vi "Initialise_puffer.vi"() -> (5 "Plug in titles":string[](array[string]), 7 "Plug in values":string[](array[string]))   [LabVIEW 2010]
uses:
  Controls/Post_Process.ctl
  ADAM Client/Sub VIs/ADAM Controls/Update_scan_value.ctl
  Globals/Meas_global.vi
  Globals/Extra_Commands_Global.vi
  Globals/Trav_pos_global.vi
  Globals/Dynamic_call_global.ph.vi
  Globals/Constants_global.vi
panel:
  out "Case Currently On":string
  out "Pulse Length":dbl format="%.2f"
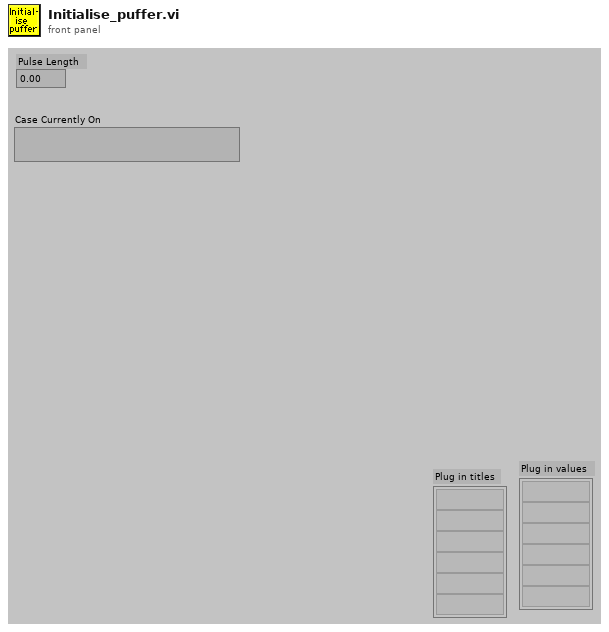
[diagram p1: front panel]
types:
  T1 = typedef "Post_Process.ctl" = enum16{"Take New Data", "Post Process Raw Data File"}
  T2 = typedef "Update_scan_value.ctl" = cluster{"Channel Name":string, "New Value":dbl}
  T3 = typedef "Traverse_cluster.ctl" = cluster{"Start X":dbl, "Start Y":dbl, "Start Z":dbl, "End X":dbl, "End Y":dbl, "End Z":dbl, "No. of pts.":i32, "Spacing":T4, "Filename":path, "Tunnel Speed":dbl, "Averaging time (min)":dbl, "Extra Commands":string, "Specific Arguments":string, "Emission Rate (l/min)":dbl, "Trace Gas Concentration (%)":dbl, "Density Ratio":string, "Comments":string, "Row No":i32, "Row Type Selector":T5, "Completion time":string, "Row Duration (mins)":dbl, "No. of Valid pts.":i32, "Meas Setup File":string}
  T4 = typedef "Spacing.ctl" = enum16{"Linear", "Log", "Gauss", "Specified", "N/A"}
  T5 = typedef "Multi_run_mode.ctl" = enum16{"Move Traverse Only", "Set Tunnel Speed Only", "Set Source Only", "Set Measurement Conditions", "Single Measurement", "Vertical Profile", "Lateral Profile", "Longitudinal Profile", "Explore Volume", "Multi-Axis Profile", "Auto Calibrate", "Meas Fast FID Bkgnd", "Check Beam Power", "Scanning Valve Measurement", "Run VI Named:", "Set ADAM Ch", "Wait (minutes)", "Send Message", "Synchronize With:", "Fall Back to this Row", "Turn Off Row Repeating", "Blank Row"}
  T6 = typedef "Rendezvous RefNum" = refnum<k1>
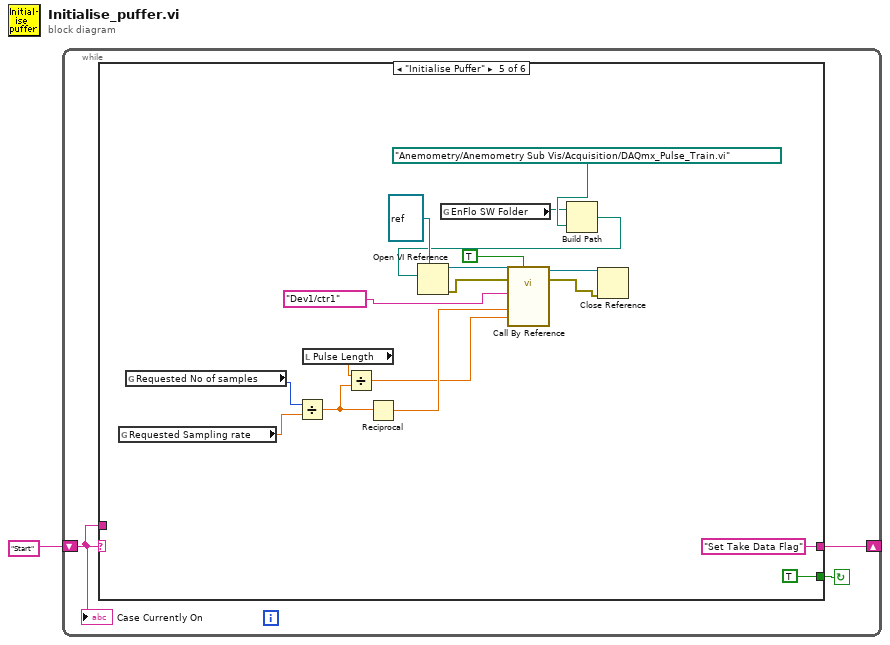
[diagram p0: block diagram]
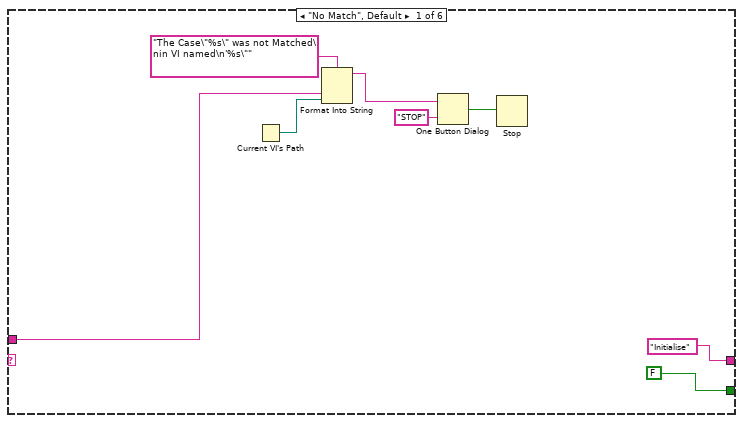
[diagram p2: hidden frame]
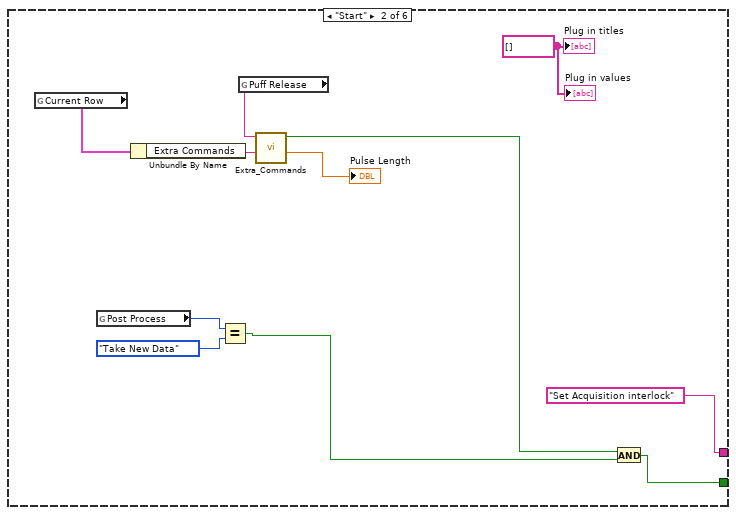
[diagram p3: hidden frame]
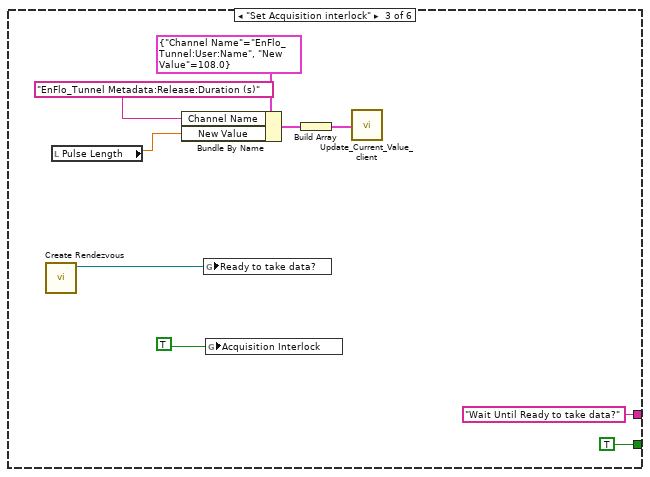
[diagram p4: hidden frame]
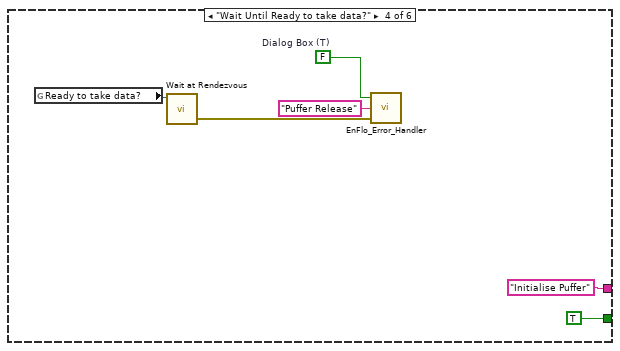
[diagram p5: hidden frame]
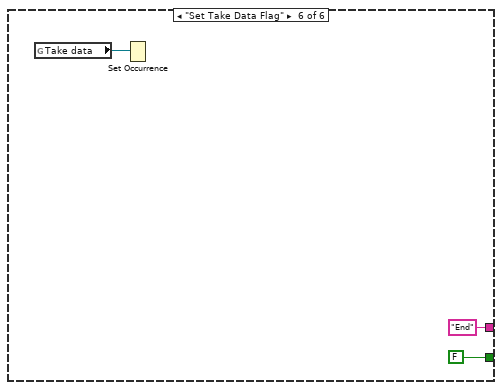
[diagram p6: hidden frame]
diagram:
  n1 = while {
    shift-left: "Start" -> [w2]
    shift-right: [w3] -> _
    stop <- w4 continue-if-true
    n2 = case shown="\"Initialise Puffer\"" w2 {
      tunnel: [FALSE w14 TRUE ("Command Found") TRUE ("Command Found") TRUE ("Command Found") FALSE ("Command Found")] -> w4
      tunnel: ["Initialise" "Set Acquisition interlock" "Wait Until Ready to take data?" "Initialise Puffer" "Set Take Data Flag" "End"] -> w3
      tunnel: w2 -> [w7 _ _ _ _ _]
      frame "No Match", Default {
        n3 = Current VI's Path() -> (path=w6:path)
        n4 = Format Into String(format string="The Case\"%s\" was not Matched\nin VI named\n'%s\"" ("Format String"), w7, w6) -> (resulting string=w10:string)  [unwired: 2 in, 1 out]
        n5 = One Button Dialog(message=w10, button name ("OK")="STOP") -> (true=w8:bool)
        n6 = Stop(stop? (T)=w8) -> ()
      }
      frame "Start" {
        w13 = string[] [] ("Plug in titles")
        n7 = global read "Trav_pos_global.vi" "Current Row"() -> (w23:T3)
        n8 = global read "Meas_global.vi" "Post Process"() -> (w17:T1)
        n9 = Unbundle By Name(w23) -> ("Extra Commands"=w21:string)
        n10 = Equal?(x=w17, y=Post_Process."Take New Data" ("Post Process")) -> (x = y?=w15:bool)
        n11 = global read "Extra_Commands_Global.vi" "Puff Release"() -> (w22:string)
        n12 = call "Extra_Commands.vi"("String to Search"=w21, "Command"=w22) -> ("Numeric Value"=→"Pulse Length":dbl, "Command Found"=w16:bool)  [unwired: 2 in, 2 out]
        n13 = And(x=w16, y=w15) -> (x .and. y?=w14:bool)
        "Plug in values" <- w13
        "Plug in titles" <- w13
      }
      frame "Set Acquisition interlock" {
        n14 = call <vilib>:"Create Rendezvous.vi"() -> ("rendezvous"=w29:T6)  [unwired: 5 in, 2 out]
        n15 = local read "Pulse Length"() -> (w24:dbl)
        n16 = Bundle By Name(cluster=T2 {"Channel Name"="EnFlo_Tunnel:User:Name", "New Value"=108.0} ("Update Scan Value Cluster"), "Channel Name"="EnFlo_Tunnel Metadata:Release:Duration (s)", "New Value"=w24) -> (w27:T2)
        n17 = global write "Dynamic_call_global.ph.vi" "Ready to take data?"(w29) -> ()
        n18 = global write "Dynamic_call_global.ph.vi" "Acquisition Interlock"(TRUE ("Remote control")) -> ()
        n19 = Build Array(w27) -> (w26:T2[])
        n20 = call "Update_Current_Value_client.vi"("Update array in"=w26) -> ()  [unwired: 1 in]
      }
      frame "Wait Until Ready to take data?" {
        w34 = FALSE  # Dialog Box (T)
        n21 = global read "Dynamic_call_global.ph.vi" "Ready to take data?"() -> (w37:T6)
        n22 = call <vilib>:"Wait at Rendezvous.vi"("rendezvous"=w37) -> ("error out"=w35:errorcluster)  [unwired: 4 in, 2 out]
        n23 = call "EnFlo_Error_Handler.vi"("error in (no error)"=w35, "Error Type"="Puffer Release", "Dialog Box (T)"=w34) -> ()  [unwired: 3 out]
      }
      frame "Initialise Puffer" {
        n24 = global read "Meas_global.vi" "Requested Sampling rate"() -> (w54:dbl)
        n25 = global read "Meas_global.vi" "Requested No of samples"() -> (w55:i32)
        n26 = Divide(x=w55, y=w54) -> (x/y=w42:dbl)
        n27 = local read "Pulse Length"() -> (w41:dbl)
        n28 = Divide(x=w41, y=w42) -> (x/y=w40:dbl)
        n29 = Reciprocal(x=w42) -> (1/x=w43:dbl)
        n30 = global read "Constants_global.vi" "EnFlo SW Folder"() -> (w45:path)
        n31 = Build Path(base path=w45, name or relative path=path "Anemometry/Anemometry Sub Vis/Acquisition/DAQmx_Pulse_Train.vi") -> (appended path=w47:path)
        n32 = Open VI Reference(type specifier VI Refnum (for type only)=refnum<vi> refnum, vi path=w47) -> (vi reference=w48:refnum<vi>, error out=w51:errorcluster)  [unwired: 4 in]
        n33 = call-by-ref "?"(reference=w48, error in=w51, "Counter(s)"=tag "Dev1/ctr1", "Start?"=TRUE, "Frequency"=w43, "Duty Cycle"=w40) -> (reference out=w50:refnum<vi>, error out=w52:errorcluster)  [unwired: 5 in]
        n34 = Close Reference(reference=w50, error in (no error)=w52) -> ()  [unwired: 1 out]
      }
      frame "Set Take Data Flag" {
        n35 = global read "Dynamic_call_global.ph.vi" "Take data"() -> (w57:refnum<k4>)
        n36 = Set Occurrence(w57) -> ()
      }
    }
    "Case Currently On" <- w2
  }
